vi "FilterConfigDataWithKeys.vi"(3 "Selected Items":string[][](array[string]), 5 "Keys":string[](array[string])) -> (1 "Filtered Selected Items":string[][](array[string]))   [LabVIEW 2018]
doc: "*-----------------------------------------------------\n* Author: SWatts\n*\n* VI Description: Filters Selected items for the list of keys\n* \n*\n* Error handling: All errors passed out\n*\n* Pre-condition: \n*\n* Post-condition: None\n*\n* Revision History:\n*\n* Rev Date Author Description \n* 01 30/04/2014 SWatts First issue\n*\n*-----------------------------------------------------"
panel:
  # "Input"
  # "Output"
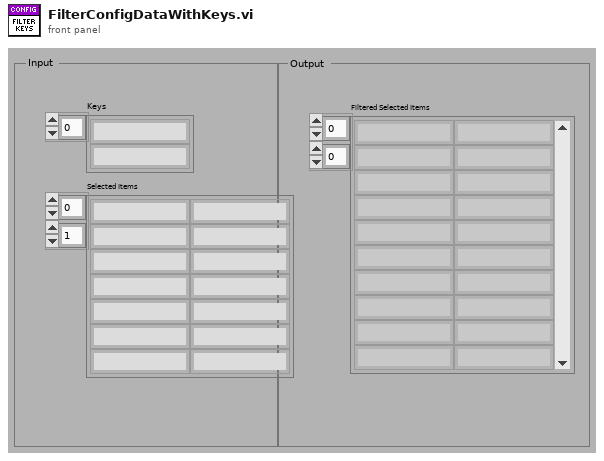
[diagram p1: front panel]
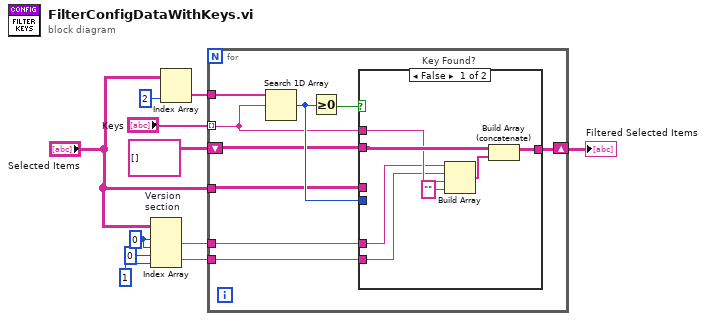
[diagram p0: block diagram]
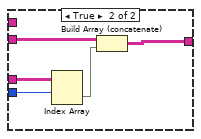
[diagram p2: hidden frame]
diagram:
  w6 = 0 ("index (row)")
  n1 = Index Array "Version\nsection"(array="Selected Items", index (row) #1=w6, index (col) #1=w6, index (row) #2=0 ("index (row)"), index (col) #2=1 ("index (row)")) -> (element #1=w5:string, element #2=w1:string)
  n2 = Index Array(array="Selected Items", index (col)=2 ("disabled index (col)")) -> (element=w9:string[])  [unwired: 1 in]
  n3 = for {
    tunnel: "Keys" -> [w14] mode=indexing
    shift-right: [w20] -> w4
    shift-left: string[][] [] ("Selected Items") -> [w17]
    tunnel: w9 -> [w16]
    tunnel: "Selected Items" -> [w18]
    tunnel: w5 -> [w13]
    tunnel: w1 -> [w12]
    n4 = Search 1D Array(1D array=w16, element=w14) -> (index of element=w19:i32)  [unwired: 1 in]
    n5 = Greater Or Equal To 0?(x=w19) -> (x >= 0?=w15:bool)
    n6 = case "Key Found?" shown="False" w15 {
      tunnel: [w26 w28] -> w20
      tunnel: w19 -> [_ w32]
      tunnel: w18 -> [_ w31]
      tunnel: w17 -> [w27 w29]
      tunnel: w14 -> [w24 _]
      tunnel: w13 -> [w22 _]
      tunnel: w12 -> [w21 _]
      frame False {
        n7 = Build Array(w22, w21, w24, "" ("element")) -> (w25:string[])
        n8 = Build Array (concatenate)(w27, w25) -> (w26:string[][])
      }
      frame True {
        n9 = Index Array(array=w31, index (row)=w32) -> (element=w30:string[])  [unwired: 1 in]
        n10 = Build Array (concatenate)(w29, w30) -> (w28:string[][])
      }
    }
  }
  "Filtered Selected Items" <- w4
